vi "运维调试_总磷总氮.vi"() -> ()   [LabVIEW 2016, in "斯坦道仪器.lvlib"]
uses:
  <vilib>/Platform/TimedLoop/XDataNode/timing_clust.ctl
  <vilib>/Platform/TimedLoop/XDataNode/nitl_modes.ctl
  <vilib>/Platform/TimedLoop/XDataNode/wakeup.ctl
  <vilib>/Utility/miscctls.llb/LVPointTypeDef.ctl
  <vilib>/Utility/config.llb/Read Key (Double).vi
  <vilib>/Utility/config.llb/Write Key (Double).vi
  <vilib>/Platform/TimedLoop/XDataNode/XDataNode.xnode
  <vilib>/Platform/TimedLoop/XDataNode/XDNodeRunTimeDep.lvlib
  <vilib>/Utility/config.llb/NI_LVConfig.lvlib
panel:
  out "字符串":string
  out "总氮稀释倍数":dbl
  out "固件版本号":string
  in  "数组":string[](array[string])
  in  "备用系数写入":bool
  in  "备用系数读取":bool
  in  "备用系数":T1
  in  "量程切换阈值写入":bool
  in  "量程切换阈值读取":bool
  in  "量程切换阈值":cluster{"阈值":dbl, "标液浓度":dbl}
  in  "参数下拉列表":enum16{"总磷", "总氮"}(ring)
  in  "量程下拉列表":enum16{"低量程", "高量程"}(ring)
  in  "测量模式下拉列表":enum16{"水样测量", "空白核查", "跨度核查", "标样核查", "加标回收"}(ring)
  in  "公式":cluster{"X^2":dbl, "X":dbl, "b":dbl}
  in  "写公式":bool
  in  "读公式":bool
  in  "精度":dbl=4.0
  in  "样品5 F0":dbl
  in  "样品5 F1":dbl
  in  "样品4 F1":dbl
  in  "样品4 F0":dbl
  in  "样品3 F0":dbl
  in  "样品3 F1":dbl
  in  "样品2 F0":dbl
  in  "样品2 F1":dbl
  in  "样品1 F1":dbl
  in  "样品1 F0":dbl
  in  "method":u16(ring) items=["最小二乘", "最小绝对残差", "Bisquare"]
  in  "模型":enum32{"线性", "多项式"}(ring)
  out "r^2":dbl format="%.7g"
  out "拟合公式":string
  in  "样品2启用":bool
  in  "样品5启用":bool
  in  "样品4启用":bool
  in  "样品3启用":bool
  in  "样品1启用":bool
  in  "标液浓度5":dbl
  out "测量吸光度5":dbl
  in  "标液浓度4":dbl
  out "测量吸光度4":dbl
  in  "标液浓度3":dbl
  out "测量吸光度3":dbl
  in  "标液浓度2":dbl
  out "测量吸光度2":dbl
  out "测量吸光度1":dbl
  in  "标液浓度1":dbl
  out "XY图":cluster{"X Values":dbl[], "Y Values":dbl[]}[](graph)
  in  "返回":bool
  in  "设置":bool
  out "序列号":string="序列号"
  out "总氮测量数据":T2(xcontrol)
  out "总磷测量数据":T2(xcontrol)
  out "集成报警信息":string
  out "设置值":dbl
  out "定时启动":bool
  out "总磷总氮运行状态":T3(xcontrol)
  in  "停止":bool
  in  "手动启动":bool
  in  "单步测试":bool
  in  "总磷氨氮调试":u16[](xcontrol)
  out "F3":sgl format="%#.6f"
  out "F2":sgl format="%#.6f"
  out "F1":sgl format="%#.6f"
  out "F0":sgl format="%#.6f"
  out "多列列表框":i32(listbox)
  # "COM5"
  # "参数设置"
  # "标液浓度"
  # "F0"
  # "F1"
  # "吸光值显示"
  # "样品一"
  # "辅\n助\n计\n算\n区"
  # "样品二"
  # "样品三"
  # "样品四"
  # "样品五"
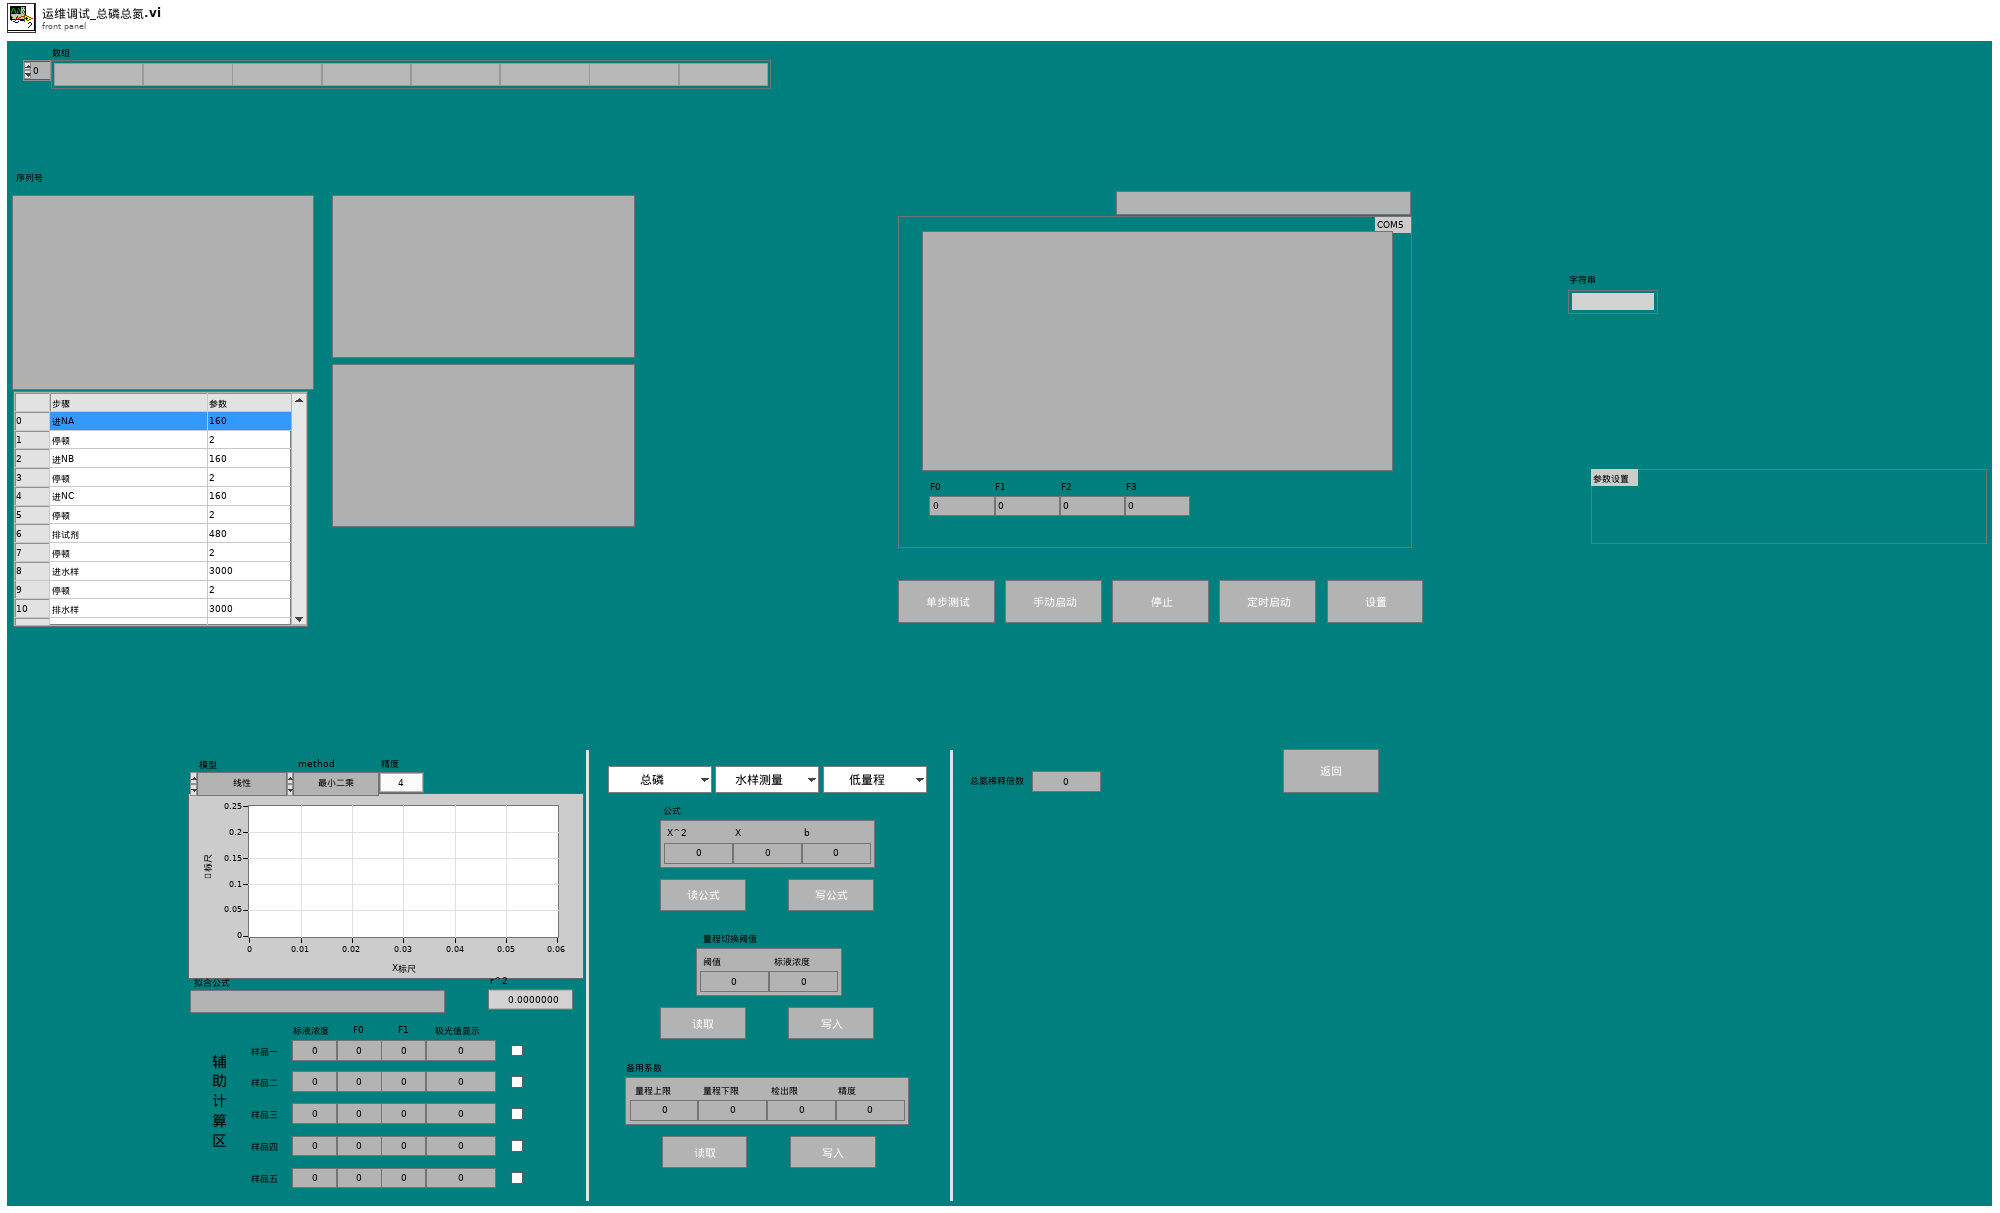
[diagram p1: front panel]
types:
  T1 = cluster{"量程上限":dbl, "量程下限":dbl, "检出限":dbl, "精度":dbl}
  T2 = cluster{"flowid":u16, "测量精度":u16, "测量数据区":cluster{"因子编码":u32, "单位":u16, "标样参考值":sgl, "水样数据时间":timestamp, "水样实测值":sgl, "水样数据标识":string, "标样数据时间":timestamp, "标样实测值":sgl, "标样数据标识":string, "空白数据时间":timestamp, "空白实测值":sgl, "空白数据标识":string, "零点核查数据时间":timestamp, "零点核查实测值":sgl, "零点核查数据标识":string, "跨度核查数据时间":timestamp, "跨度核查实测值":sgl, "跨度核查数据标识":string, "加标回收数据时间":timestamp, "加标回收实测值":sgl, "加标回收数据标识":string, "平行样数据时间":timestamp, "平行样实测值":sgl, "平行样数据标识":string, "F0":sgl, "F1":sgl, "F2":sgl, "F3":sgl, "F4":sgl, "F5":sgl, "F6":sgl, "F7":sgl, "温度":sgl, "湿度":sgl, "X值":sgl}}
  T3 = cluster{"系统时间":timestamp, "工作状态":enum16{"空闲", "水样测试", "标样核查", "零点核查", "跨度核查", "空白测试", "平行样测试", "加标回收", "空白校准", "标样校准", "初始化（清洗）"}, "测量模式":enum16{"待机", "连续模式", "周期模式", "定点模式", "受控模式", "手动模式"}, "告警代码":enum16{"无告警", "缺试剂告警", "缺水样告警", "缺蒸馏水告警", "缺标液告警", "仪表漏液告警", "标定异常告警", "超量程告警", "加热异常", "低试剂预警", "超上限告警", "超下限告警", "仪表内部其他异常", "滴定异常告警", "电极异常告警", "量程切换告警", "参数设置告警", "PH电极电位异常", "电导率电极异常", "浊度光度异常", "溶解氧电极异常", "溶解氧光强异常", "温度异常告警", "PH异常告警", "溶解氧异常告警", "电导率异常告警", "浊度异常告警", "叶绿素异常告警", "藻密度异常告警", "蓝绿藻异常告警", "ORP异常告警", "氨氮异常告警", "清洁刷异常告警", "SD卡异常告警", "蓝牙异常告警", "Wifi异常告警", "流程异常告警"}, "故障代码":enum16{"无故障", "电机故障", "温度故障", "通讯故障", "滴定故障"}, "日志代码":u16, "软件版本":u16, "F0":sgl, "F1":sgl, "F2":sgl, "F3":sgl, "T":sgl, "H":sgl, "id":u16, "flowid":u16, "量程":u16}
  T4 = enum16{"待机", "启动氨氮", "氨氮测量中", "启动总磷", "总磷测量中", "延时"}
  T5 = typedef "LVPointTypeDef.ctl" = cluster{"Horizontal":i16, "Vertical":i16}
  T6 = cluster{"因子编码":u32, "单位":u16, "标样参考值":sgl, "水样数据时间":timestamp, "水样实测值":sgl, "水样数据标识":string, "标样数据时间":timestamp, "标样实测值":sgl, "标样数据标识":string, "空白数据时间":timestamp, "空白实测值":sgl, "空白数据标识":string, "零点核查数据时间":timestamp, "零点核查实测值":sgl, "零点核查数据标识":string, "跨度核查数据时间":timestamp, "跨度核查实测值":sgl, "跨度核查数据标识":string, "加标回收数据时间":timestamp, "加标回收实测值":sgl, "加标回收数据标识":string, "平行样数据时间":timestamp, "平行样实测值":sgl, "平行样数据标识":string, "F0":sgl, "F1":sgl, "F2":sgl, "F3":sgl, "F4":sgl, "F5":sgl, "F6":sgl, "F7":sgl, "温度":sgl, "湿度":sgl, "X值":sgl}
  T7 = enum16{"空闲", "水样测试", "标样核查", "零点核查", "跨度核查", "空白测试", "平行样测试", "加标回收", "空白校准", "标样校准", "初始化（清洗）"}
  T8 = typedef "XDNodeRunTimeDep.lvlib/timing_clust.ctl" = cluster{"Expected End [f-1]":u64, "Actual End [f-1]":u64, "Finished Late? [f-1]":bool, "Expected End [i-1]":u64, "Actual End [i-1]":u64, "Finished Late? [i-1]":bool, "Expected Start [i]":u64, "Actual Start [i]":u64, "Expected Start [f]":u64, "Actual Start [f]":u64, "Source Name":string, "Structure Name":string, "Period":i64, "Deadline":i64, "Offset":i64, "Start":i64, "Priority":i32, "Timeout":i32, "Mode":T9, "Wakeup Reason":T10, "Error":errorcluster, "Source Type":string, "Secondary Source Type":string, "Global End Time":u64, "Global Start Time":u64, "Frame Duration":u64, "Iteration Duration":u64, "Assigned CPU":i32, "I/O Scan Engine Mode":u32}
  T9 = typedef "XDNodeRunTimeDep.lvlib/nitl_modes.ctl" = enum32{"No Change", "Process missed periods, maintain original phase", "Discard missed periods, maintain original phase", "Process missed periods, ignore original phase", "Discard missed periods, ignore original phase"}
  T10 = typedef "XDNodeRunTimeDep.lvlib/wakeup.ctl" = enum32{"Normal", "Aborted", "Asynchronous wakeup", "Timing source error", "Timed loop error", "Timeout"}
  T11 = cluster{"启动模式":enum16{"标液测量", "水样测量", "零液测量", "盲样测量", "加标回收"}, "启动参数":u16, "量程":enum16{"低量程", "高量程"}}
  T12 = cluster{"时间标识":timestamp, "设备":string, "日志信息":string, "流程参数":string}
  T13 = cluster{"时间标识":timestamp, "设备":string, "日志信息":string}
  T14 = enum16{"无告警", "缺试剂告警", "缺水样告警", "缺蒸馏水告警", "缺标液告警", "仪表漏液告警", "标定异常告警", "超量程告警", "加热异常", "低试剂预警", "超上限告警", "超下限告警", "仪表内部其他异常", "滴定异常告警", "电极异常告警", "量程切换告警", "参数设置告警", "PH电极电位异常", "电导率电极异常", "浊度光度异常", "溶解氧电极异常", "溶解氧光强异常", "温度异常告警", "PH异常告警", "溶解氧异常告警", "电导率异常告警", "浊度异常告警", "叶绿素异常告警", "藻密度异常告警", "蓝绿藻异常告警", "ORP异常告警", "氨氮异常告警", "清洁刷异常告警", "SD卡异常告警", "蓝牙异常告警", "Wifi异常告警", "流程异常告警"}
  T15 = typedef "LVRowAndColumnUnsignedTypeDef.ctl" = cluster{"Row":u32, "Column":u32}
  T16 = typedef "NI_LVConfig.lvlib/Config Data RefNum.ctl" = refnum<k1>
  T17 = cluster{"站号":u16, "量程切换":enum32{"H", "L", "AUTO"}, "控制命令":enum16{"启动测量", "标样核查", "零点核查", "跨度核查", "空白测试", "平行样测试", "加标回收", "空白校准", "标样校准", "初始化（清洗）", "停止测试", "仪器重启", "校时", "模式设置", "测量间隔设置", "盲样测试"}, "模式设置":enum16{"待机", "连续模式", "周期模式", "定点模式", "受控模式", "手动模式"}, "测量间隔":u16}
  T18 = cluster{"站号":u16, "量程切换":enum32{"H", "L", "AUTO"}, "控制命令":enum16{"启动测量", "标样核查", "零点核查", "跨度核查", "空白测试", "平行样测试", "加标回收", "空白校准", "标样校准", "初始化（清洗）", "停止测试", "仪器重启", "校时", "模式设置", "测量间隔设置"}, "模式设置":enum16{"待机", "连续模式", "周期模式", "定点模式", "受控模式", "手动模式"}, "测量间隔":u16}
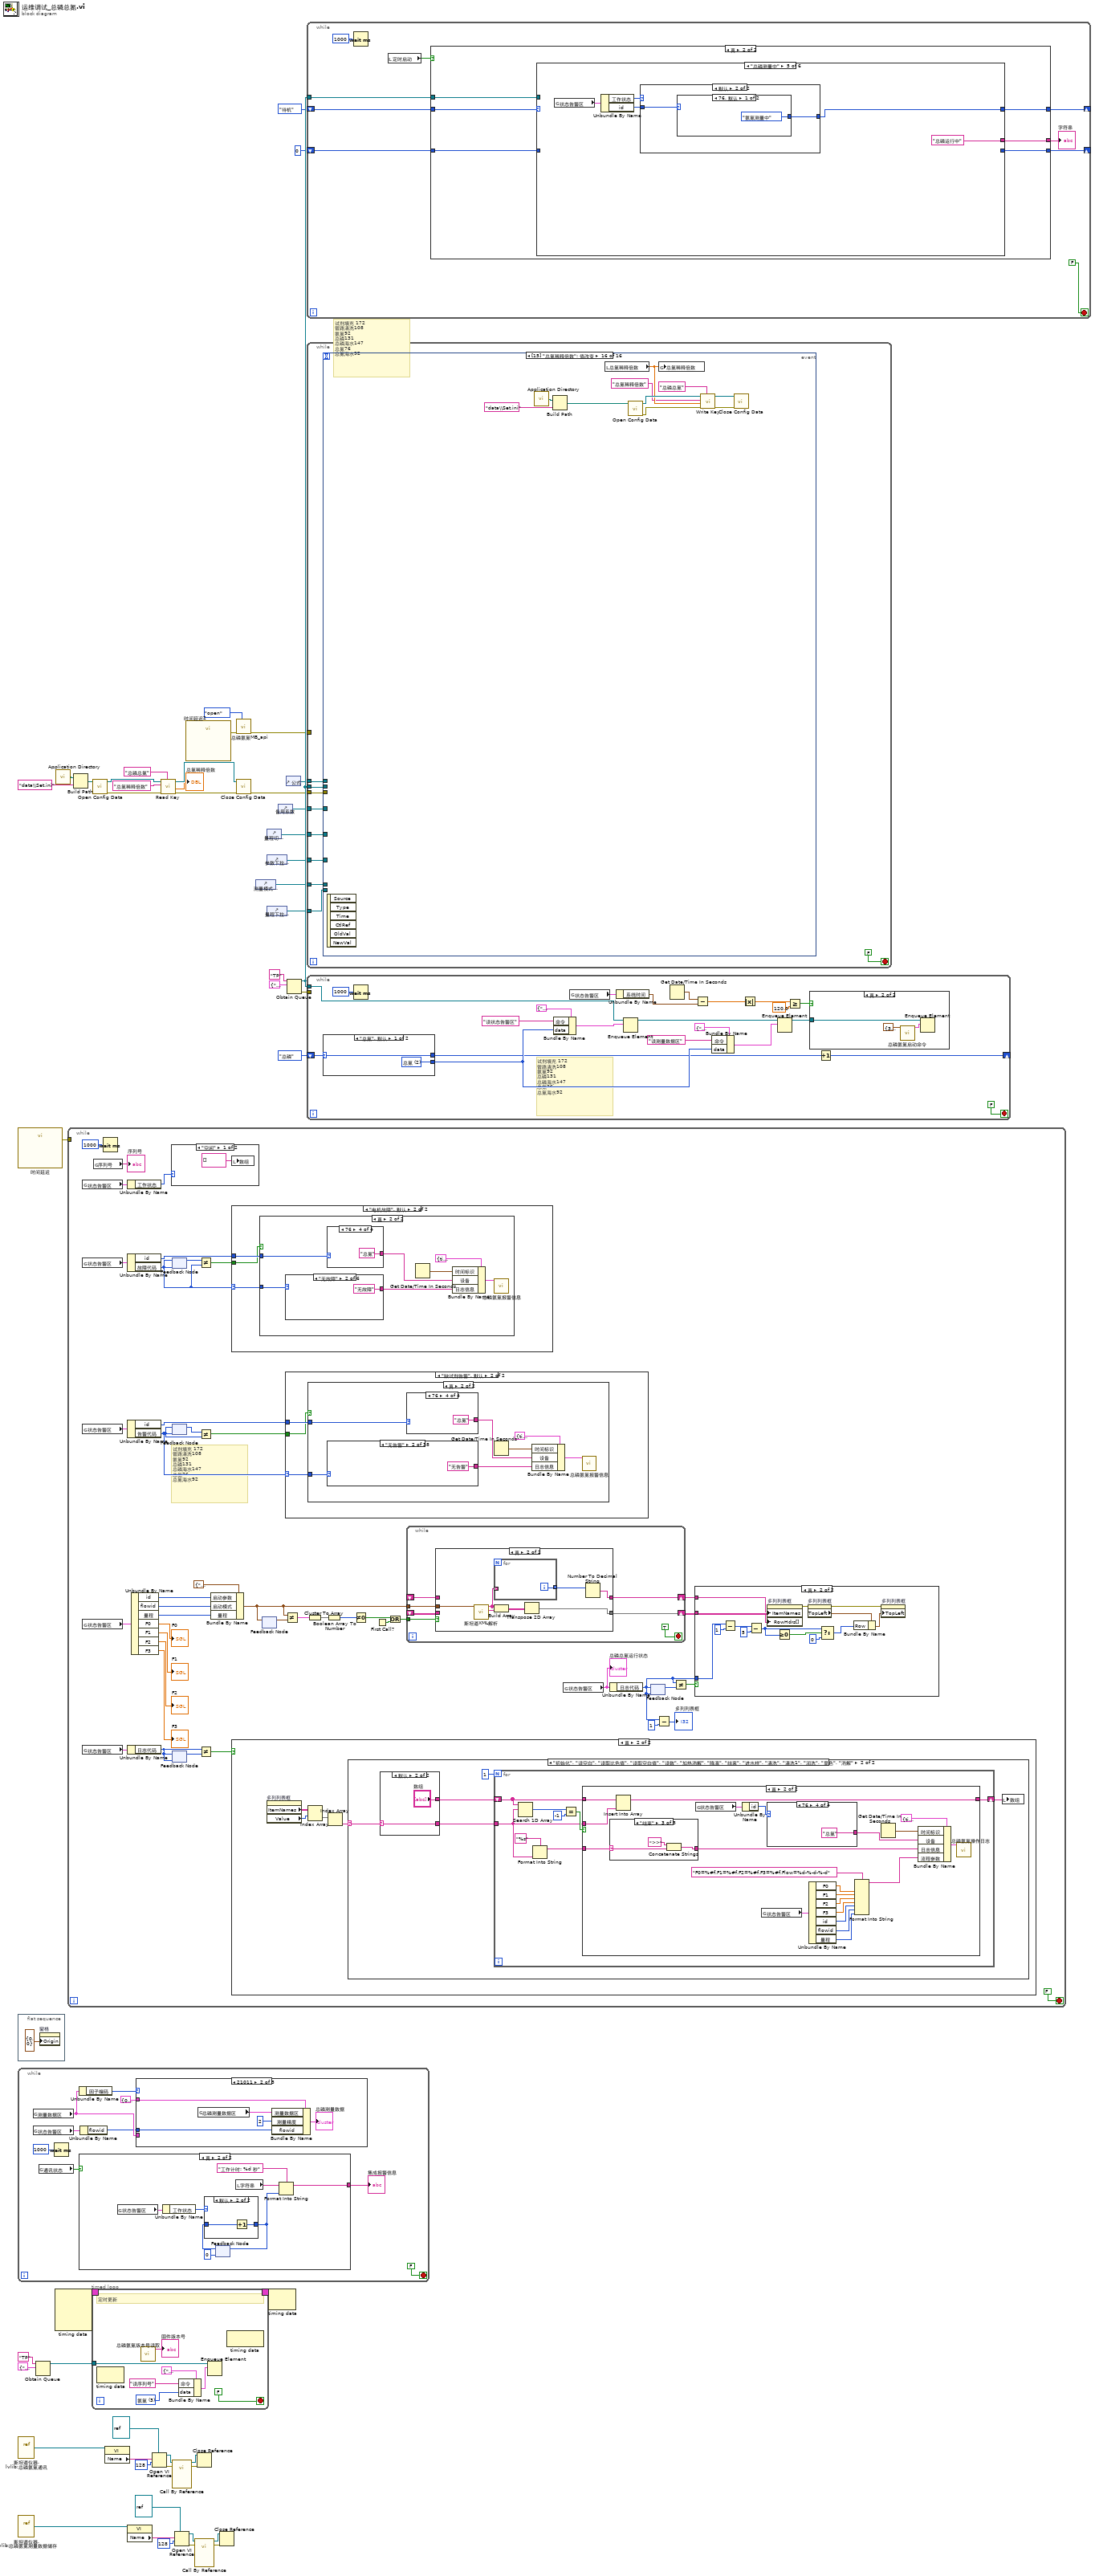
[diagram p0: block diagram]
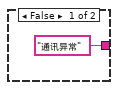
[diagram p2: hidden frame]
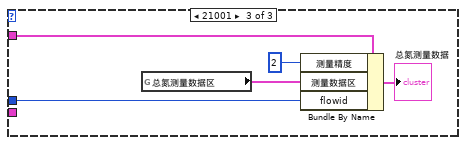
[diagram p5: hidden frame]
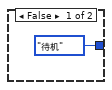
[diagram p6: hidden frame]
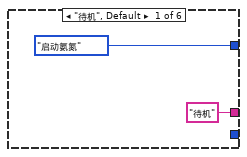
[diagram p7: hidden frame]
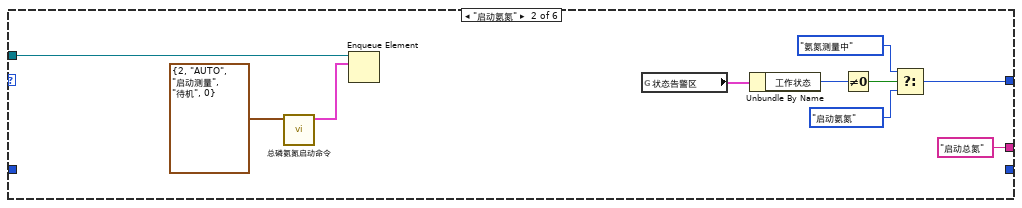
[diagram p8: hidden frame]
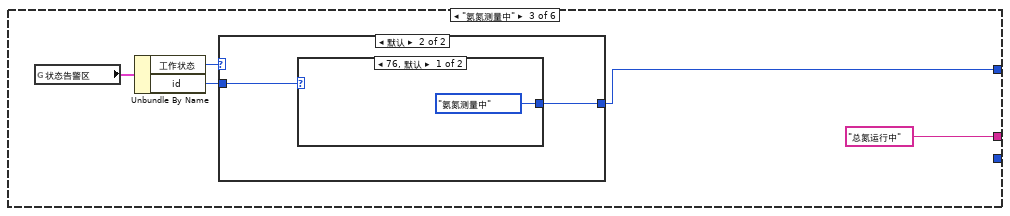
[diagram p9: hidden frame]
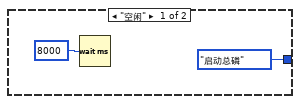
[diagram p10: hidden frame]
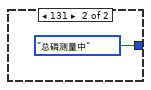
[diagram p11: hidden frame]
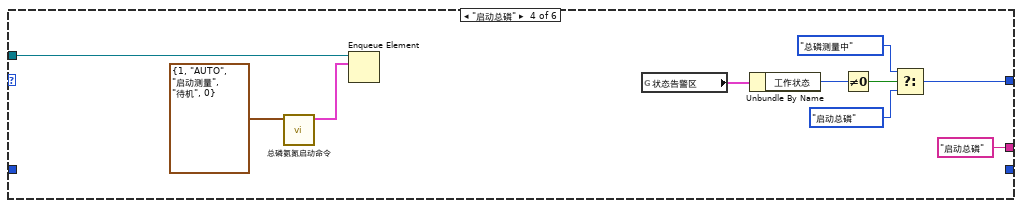
[diagram p12: hidden frame]
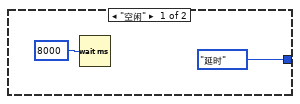
[diagram p13: hidden frame]
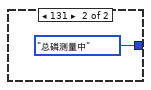
[diagram p14: hidden frame]
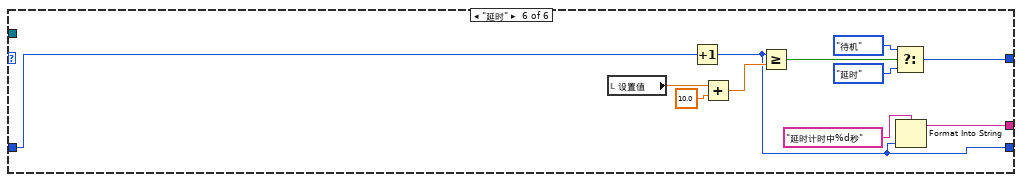
[diagram p15: hidden frame]
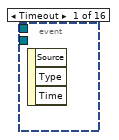
[diagram p16: hidden frame]
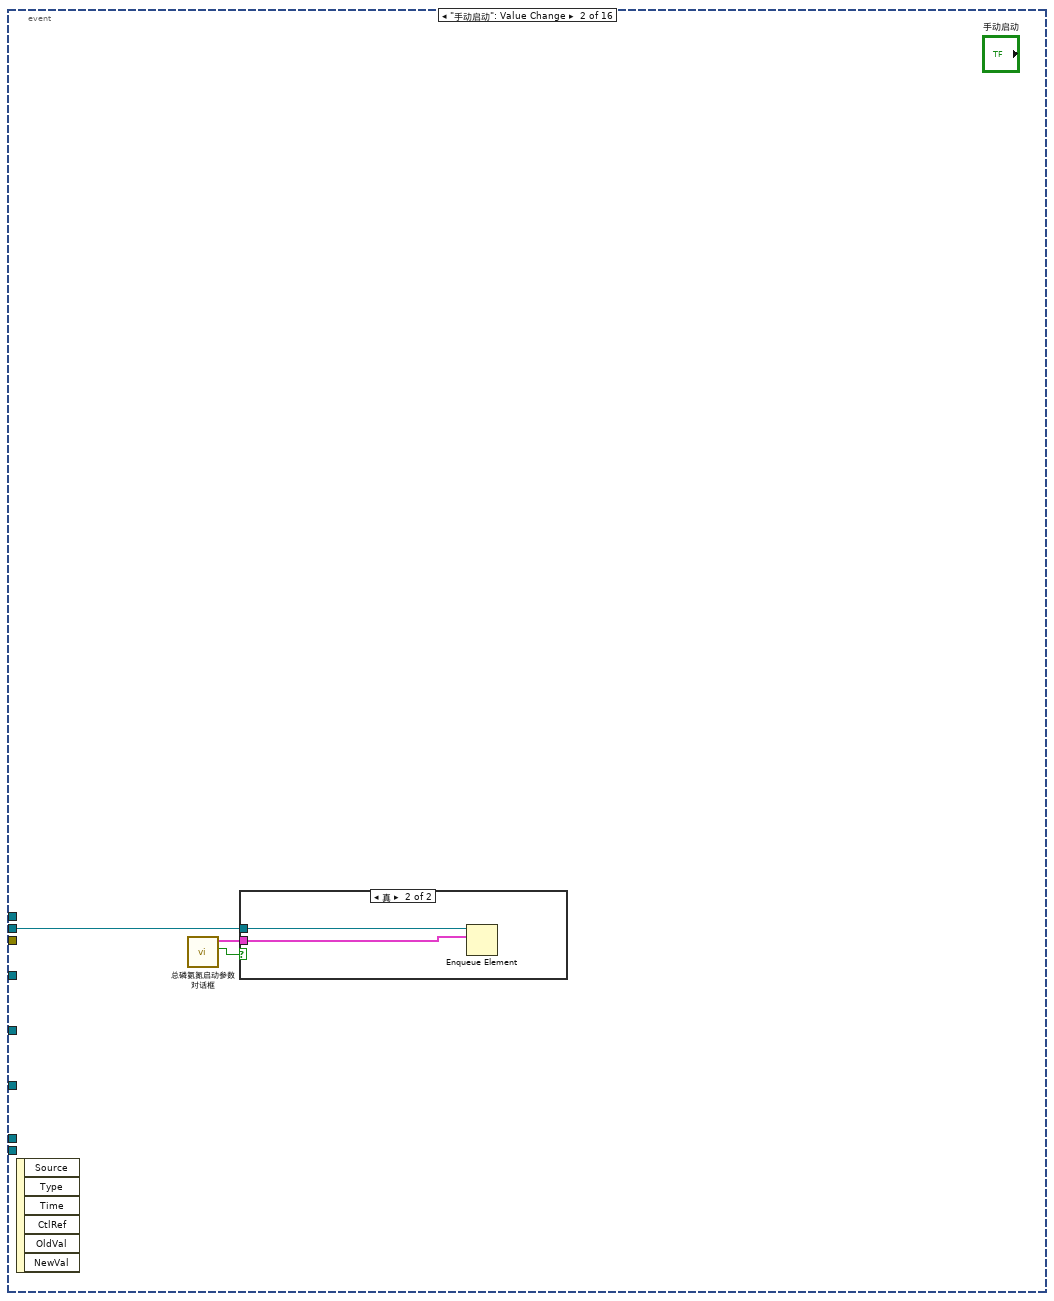
[diagram p17: hidden frame]
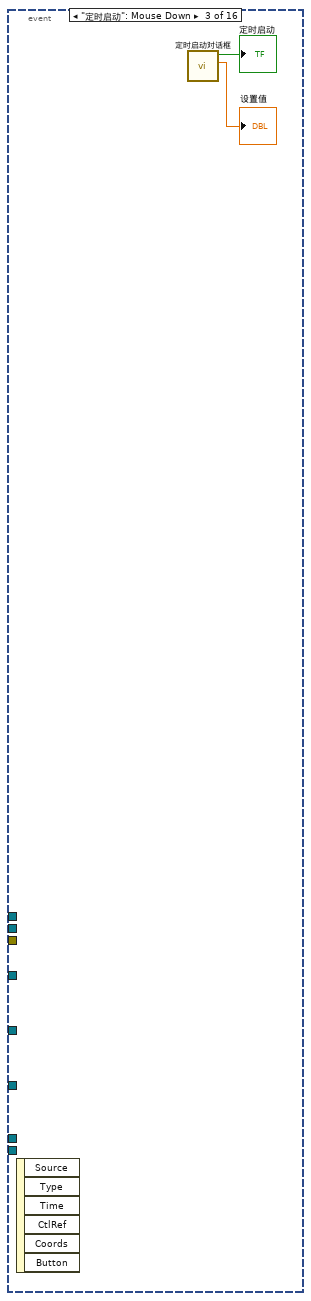
[diagram p19: hidden frame]
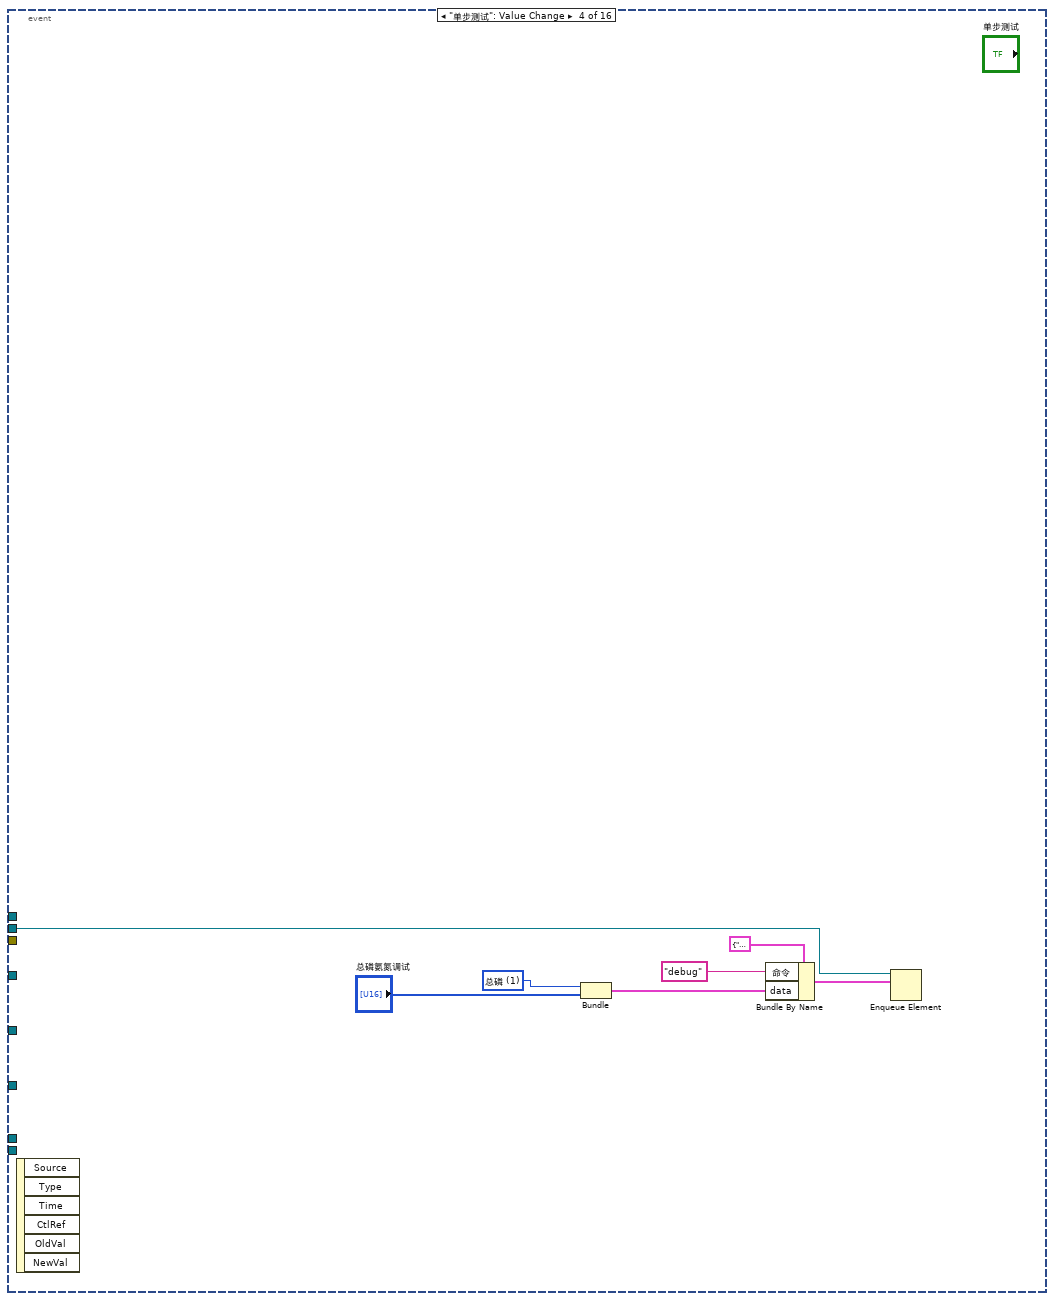
[diagram p20: hidden frame]
diagram:
  # "试剂填充 172 \n管路清洗108\n氨氮92\n总磷131\n总磷海水147\n总氮76\n总氮海水92"
  n1 = call "时间延迟"() -> ("error out"=w20:errorcluster)  [unwired: 11 in]
  n2 = flat-sequence {
    frame #0 {
      n3 = property on="窗格" class="Pane"("Origin"=T5 {"Horizontal"=0, "Vertical"=0} ("原点")) -> ()  [unwired: 2 in, 2 out]
    }
  }
  n4 = while {
    stop <- FALSE stop-if-true
    n5 = global read "VAR总磷氨氮全局变量.vi" "测量数据区"() -> (w57:T6)
    n6 = global read "VAR总磷氨氮全局变量.vi" "状态告警区"() -> (w53:T3)
    n7 = global read "VAR总磷氨氮全局变量.vi" "通讯状态"() -> (w55:bool)
    n8 = Wait (ms)(milliseconds to wait=u32 1000 ("等待时间（毫秒）")) -> ()  [unwired: 1 out]
    n9 = Unbundle By Name(w57) -> ("因子编码"=w56:u32)
    n10 = case shown="真" w55 {
      tunnel: ["通讯异常" ("集成报警信息") w62] -> w54
      frame False {
      }
      frame True {
        n11 = global read "VAR总磷氨氮全局变量.vi" "状态告警区"() -> (w68:T3)
        n12 = Unbundle By Name(w68) -> ("工作状态"=w67:T7)
        n13 = feedback #1(0) -> (w65:i32)
        n14 = case shown="默认" w67 {
          tunnel: w65 -> [_ w70]
          tunnel: [_ w69] -> w63
          frame "空闲" {
          }
          frame Default {
            n15 = Increment(x=w70) -> (x+1=w69:i32)
          }
        }
        n16 = feedback-in #1(w63) -> ()
        n17 = local read "字符串"() -> (w61:string)
        n18 = Format Into String(format string="工作计时: %d 秒" ("格式字符串"), initial string=w61, w63) -> (resulting string=w62:string)  [unwired: 1 in, 1 out]
      }
    }
    "集成报警信息" <- w54
    n19 = Unbundle By Name(w53) -> ("flowid"=w52:u16)
    n20 = case shown="21011" w56 {
      tunnel: w57 -> [_ _ _]
      tunnel: w52 -> [_ w73 w79]
      tunnel: T2 {"flowid"=0, "测量精度"=0, "测量数据区"={"因子编码"=0, "单位"=0, "标样参考值"=0.0, "水样数据时间"=timestamp(0 s since 1904-01-01), "水样实测值"=0.0, "水样数据标识"="", "标样数据时间"=timestamp(0 s since 1904-01-01), "标样实测值"=0.0, "标样数据标识"="", "空白数据时间"=timestamp(0 s since 1904-01-01), "空白实测值"=0.0, "空白数据标识"="", "零点核查数据时间"=timestamp(0 s since 1904-01-01), "零点核查实测值"=0.0, "零点核查数据标识"="", "跨度核查数据时间"=timestamp(0 s since 1904-01-01), "跨度核查实测值"=0.0, "跨度核查数据标识"="", "加标回收数据时间"=timestamp(0 s since 1904-01-01), "加标回收实测值"=0.0, "加标回收数据标识"="", "平行样数据时间"=timestamp(0 s since 1904-01-01), "平行样实测值"=0.0, "平行样数据标识"="", "F0"=0.0, "F1"=0.0, "F2"=0.0, "F3"=0.0, "F4"=0.0, "F5"=0.0, "F6"=0.0, "F7"=0.0, "温度"=0.0, "湿度"=0.0, "X值"=0.0}} ("总氮测量数据") -> [_ w72 w78]
      frame Default {
      }
      frame 21011 {
        n21 = global read "VAR总磷氨氮全局变量.vi" "总磷测量数据区"() -> (w71:T6)
        n22 = Bundle By Name(cluster=w72, "测量数据区"=w71, "测量精度"=u16 2, "flowid"=w73) -> (→"总磷测量数据":T2)
      }
      frame 21001 {
        n23 = global read "VAR总磷氨氮全局变量.vi" "总氮测量数据区"() -> (w76:T6)
        n24 = Bundle By Name(cluster=w78, "测量精度"=u16 2, "测量数据区"=w76, "flowid"=w79) -> (→"总氮测量数据":T2)
      }
    }
  }
  n25 = vi-ref "斯坦道仪器.lvlib:总磷氨氮通讯.vi"() -> (w43:refnum<vi>)
  n26 = vi-ref "斯坦道仪器.lvlib:总磷氨氮测量数据储存.vi"() -> (w35:refnum<vi>)
  n27 = Obtain Queue(name (unnamed)="TP" ("名称（未命名）"), element data type=cluster{"命令":string, "data":variant} {"命令"="", "data"=variant}) -> (queue out=w13:refnum<queue>)  [unwired: 3 in, 2 out]
  n28 = node-c288() -> (w17:T8)  [unwired: 4 in]
  n29 = call <vilib>:"Application Directory.vi"() -> ("Application Directory"=w7:path)
  n30 = while {
    tunnel: w20 -> [_]
    stop <- FALSE stop-if-true
    # "试剂填充 172 \n管路清洗108\n氨氮92\n总磷131\n总磷海水147\n总氮76\n总氮海水92"
    n31 = global read "VAR总磷氨氮全局变量.vi" "状态告警区"() -> (w89:T3)
    n32 = global read "VAR总磷氨氮全局变量.vi" "状态告警区"() -> (w94:T3)
    n33 = global read "VAR总磷氨氮全局变量.vi" "状态告警区"() -> (w99:T3)
    n34 = global read "VAR总磷氨氮全局变量.vi" "状态告警区"() -> (w111:T3)
    n35 = global read "VAR总磷氨氮全局变量.vi" "状态告警区"() -> (w86:T3)
    n36 = global read "VAR总磷氨氮全局变量.vi" "序列号"() -> (→"序列号":string)
    n37 = Wait (ms)(milliseconds to wait=u32 1000 ("等待时间（毫秒）")) -> ()  [unwired: 1 out]
    n38 = Unbundle By Name(w89) -> ("工作状态"=w88:T7)
    n39 = Unbundle By Name(w94) -> ("id"=w93:u16, "故障代码"=w90:enum16{"无故障", "电机故障", "温度故障", "通讯故障", "滴定故障"})
    n40 = Unbundle By Name(w99) -> ("id"=w98:u16, "告警代码"=w95:T14)
    n41 = Unbundle By Name(w86) -> ("日志代码"=w85:u16)
    n42 = Unbundle By Name(w111) -> ("id"=w108:u16, "flowid"=w110:u16, "量程"=w109:u16, "F0"=→"F0":sgl, "F1"=→"F1":sgl, "F2"=→"F2":sgl, "F3"=→"F3":sgl)
    n43 = case shown="\"空闲\"" w88 {
      frame "空闲" {
        n44 = local write "数组"(string[] [] ("数组")) -> ()
      }
      frame "水样测试", Default {
      }
    }
    n45 = feedback #2(w90) -> (w91:enum16{"无故障", "电机故障", "温度故障", "通讯故障", "滴定故障"})
    n46 = feedback-in #2(w90) -> ()
    n47 = feedback #3(w95) -> (w96:T14)
    n48 = feedback-in #3(w95) -> ()
    n49 = feedback #4(w85) -> (w87:u16)
    n50 = feedback-in #4(w85) -> ()
    n51 = Not Equal?(x=w91, y=w90) -> (x != y?=w92:bool)
    n52 = Not Equal?(x=w96, y=w95) -> (x != y?=w97:bool)
    n53 = Not Equal?(x=w85, y=w87) -> (x != y?=w84:bool)
    n54 = Bundle By Name(cluster=T11 {"启动模式"=enum."加标回收", "启动参数"=1, "量程"=enum."低量程"} ("参数簇"), "启动参数"=w108, "启动模式"=w110, "量程"=w109) -> (w101:T11)
    n55 = case shown="\"电机故障\", 默认" w90 {
      selector: w90 -> [_ w180]
      tunnel: w93 -> [_ w181]
      tunnel: w92 -> [_ w179]
      frame "无故障" {
      }
      frame "电机故障", Default {
        n56 = case shown="真" w179 {
          tunnel: w181 -> [_ w188]
          tunnel: w180 -> [_ w183]
          frame False {
          }
          frame True {
            n57 = case shown="\"无故障\"" w183 {
              selector: w183 -> [w190 _ _ _ _ _]
              tunnel: [w189 "无故障" "电机故障" "温度故障" "通讯故障" "滴定故障"] -> w182
              frame Default {
                n58 = Format Into String(format string="%d" ("格式字符串"), initial string="未知" ("工作状态"), w190) -> (resulting string=w189:string)  [unwired: 1 in, 1 out]
              }
              frame "无故障" {
              }
              frame "电机故障" {
              }
              frame "温度故障" {
              }
              frame "通讯故障" {
              }
              frame "滴定故障" {
              }
            }
            n59 = case shown="76" w188 {
              tunnel: [_ "总磷" ("table输入") "氨氮" ("table输入") "总氮" ("table输入")] -> w184
              frame Default {
              }
              frame 131 {
              }
              frame 92 {
              }
              frame 76 {
              }
            }
            n60 = Get Date/Time In Seconds() -> (seconds since 1Jan1904=w185:timestamp)
            n61 = Bundle By Name(cluster=T13 {"时间标识"=timestamp(0 s since 1904-01-01), "设备"="", "日志信息"=""} ("data in"), "时间标识"=w185, "设备"=w184, "日志信息"=w182) -> (w186:T13)
            n62 = call "总磷氨氮报警信息.vi"("data in"=w186) -> ()  [unwired: 11 in]
          }
        }
      }
    }
    n63 = case shown="真" w84 {
      frame False {
      }
      frame True {
        n64 = property on="多列列表框" class="MCListbox (严格)"() -> ("ItemNames"=w128:string[][], "Value"=w129:i32)  [unwired: 2 in, 2 out]
        n65 = Index Array(array=w128, index (row)=w129) -> (element=w127:string[])  [unwired: 1 in]
        n66 = Index Array(array=w127) -> (element=w126:string)  [unwired: 1 in]
        n67 = case shown="\"初始化\", \"读空白\", \"读取比色值\", \"读取空白值\", \"读数\", \"加热消解\", \"降温\", \"结束\", \"进水样\", \"清洗\", \"清洗1\", \"润洗\", \"显色\", \"消解\"" w126 {
          selector: w126 -> [_ w132]
          frame Default {
          }
          frame "初始化", "读空白", "读取比色值", "读取空白值", "读数", "加热消解", "降温", "结束", "进水样", "清洗", "清洗1", "润洗", "显色", "消解" {
            n68 = case shown="默认" w132 {
              selector: w132 -> [w136 w138]
              tunnel: [w136 w138] -> w131
              tunnel: [string[] [] ("数组") "数组"] -> w130
              frame "读数" {
              }
              frame Default {
              }
            }
            n69 = for {
              N: 1 -> [_]
              tunnel: w131 -> [w140]
              shift-right: [w139] -> w133
              shift-left: w130 -> [w141]
              n70 = Search 1D Array(1D array=w141, element=w140) -> (index of element=w144:i32)  [unwired: 1 in]
              n71 = Format Into String(format string="%s" ("格式字符串"), w140) -> (resulting string=w145:string)  [unwired: 2 in, 1 out]
              n72 = Equal?(x=w144, y=-1) -> (x = y?=w142:bool)
              n73 = case shown="真" w142 {
                tunnel: w145 -> [_ w149]
                tunnel: w141 -> [w147 w153]
                tunnel: w140 -> [_ w152]
                tunnel: [w147 w151] -> w139
                frame False {
                }
                frame True {
                  n74 = case shown="\"结束\"" w149 {
                    selector: w149 -> [w169 w172 w175]
                    tunnel: [w169 w171 w174] -> w148
                    frame Default {
                    }
                    frame "初始化" {
                      n75 = Concatenate Strings("<<" ("字符串"), w172) -> (w171:string)
                    }
                    frame "结束" {
                      n76 = Concatenate Strings(">>" ("字符串"), w175) -> (w174:string)
                    }
                  }
                  n77 = Insert Into Array(array=w153, new element=w152) -> (w151:string[])  [unwired: 1 in]
                  n78 = global read "VAR总磷氨氮全局变量.vi" "状态告警区"() -> (w168:T3)
                  n79 = Unbundle By Name(w168) -> ("id"=w167:u16)
                  n80 = global read "VAR总磷氨氮全局变量.vi" "状态告警区"() -> (w163:T3)
                  n81 = case shown="76" w167 {
                    tunnel: [_ "总磷" ("table输入") "氨氮" ("table输入") "总氮" ("table输入")] -> w165
                    frame Default {
                    }
                    frame 131 {
                    }
                    frame 92 {
                    }
                    frame 76 {
                    }
                  }
                  n82 = Unbundle By Name(w163) -> ("F0"=w160:sgl, "F1"=w159:sgl, "F2"=w158:sgl, "F3"=w157:sgl, "id"=w156:u16, "flowid"=w155:u16, "量程"=w154:u16)
                  n83 = Format Into String(format string="F0=%#f,F1=%#f,F2=%#f,F3=%#f,Flow=%d-%-d-%-d" ("格式字符串"), w160, w159, w158, w157, w156, w155, w154) -> (resulting string=w161:string)  [unwired: 2 in, 1 out]
                  n84 = Get Date/Time In Seconds() -> (seconds since 1Jan1904=w164:timestamp)
                  n85 = Bundle By Name(cluster=T12 {"时间标识"=timestamp(0 s since 1904-01-01), "设备"="", "日志信息"="", "流程参数"=""} ("data in"), "时间标识"=w164, "设备"=w165, "日志信息"=w148, "流程参数"=w161) -> (w166:T12)
                  n86 = call "总磷氨氮操作日志.vi"("data in"=w166) -> ()  [unwired: 11 in]
                }
              }
            }
            n87 = local write "数组"(w133) -> ()
          }
        }
      }
    }
    n88 = feedback #5() -> (w117:T11)  [unwired: 1 in]
    n89 = feedback-in #5(w101) -> ()
    n90 = Not Equal?(x=w101, y=w117) -> (x != y?=w118:cluster{"启动模式":bool, "启动参数":bool, "量程":bool})
    n91 = case shown="\"缺试剂告警\", 默认" w95 {
      selector: w95 -> [_ w202]
      tunnel: w98 -> [_ w203]
      tunnel: w97 -> [_ w201]
      frame "无告警" {
      }
      frame "缺试剂告警", Default {
        n92 = case shown="真" w201 {
          tunnel: w203 -> [_ w210]
          tunnel: w202 -> [_ w204]
          frame False {
          }
          frame True {
            n93 = case shown="\"无告警\"" w204 {
              selector: w204 -> [w212 _ _ _ _ _ _ _ _ _ _ _ _ _ _ _ _ _ _ _ _ _ _ _ _ _ _ _ _ _ _ _ _ _ _ _ _ _]
              tunnel: [w211 "无告警" "缺试剂告警" "缺水样告警" "缺蒸馏水告警" "缺标液告警" "仪表漏液告警" "标定异常告警" "超量程告警" "加热异常" "低试剂预警" "超上限告警" "超下限告警" "仪表内部其他异常" "滴定异常告警" "电极异常告警" "量程切换告警" "参数设置告警" "PH电极电位异常" "电导率电极异常" "浊度光度异常" "溶解氧电极异常" "溶解氧光强异常" "温度异常告警" "PH异常告警" "溶解氧异常告警" "电导率异常告警" "浊度异常告警" "叶绿素异常告警" "藻密度异常告警" "蓝绿藻异常告警" "ORP异常告警" "氨氮异常告警" "清洁刷异常告警" "SD卡异常告警" "蓝牙异常告警" "WiFi异常告警" "流程异常告警"] -> w205
              frame Default {
                n94 = Format Into String(format string="%d" ("格式字符串"), initial string="未知" ("工作状态"), w212) -> (resulting string=w211:string)  [unwired: 1 in, 1 out]
              }
              frame "无告警" {
              }
              frame "缺试剂告警" {
              }
              frame "缺水样告警" {
              }
              frame "缺蒸馏水告警" {
              }
              frame "缺标液告警" {
              }
              frame "仪表漏液告警" {
              }
              frame "标定异常告警" {
              }
              frame "超量程告警" {
              }
              frame "加热异常" {
              }
              frame "低试剂预警" {
              }
              frame "超上限告警" {
              }
              frame "超下限告警" {
              }
              frame "仪表内部其他异常" {
              }
              frame "滴定异常告警" {
              }
              frame "电极异常告警" {
              }
              frame "量程切换告警" {
              }
              frame "参数设置告警" {
              }
              frame "PH电极电位异常" {
              }
              frame "电导率电极异常" {
              }
              frame "浊度光度异常" {
              }
              frame "溶解氧电极异常" {
              }
              frame "溶解氧光强异常" {
              }
              frame "温度异常告警" {
              }
              frame "PH异常告警" {
              }
              frame "溶解氧异常告警" {
              }
              frame "电导率异常告警" {
              }
              frame "浊度异常告警" {
              }
              frame "叶绿素异常告警" {
              }
              frame "藻密度异常告警" {
              }
              frame "蓝绿藻异常告警" {
              }
              frame "ORP异常告警" {
              }
              frame "氨氮异常告警" {
              }
              frame "清洁刷异常告警" {
              }
              frame "SD卡异常告警" {
              }
              frame "蓝牙异常告警" {
              }
              frame "Wifi异常告警" {
              }
              frame "流程异常告警" {
              }
            }
            n95 = case shown="76" w210 {
              tunnel: [_ "总磷" ("table输入") "氨氮" ("table输入") "总氮" ("table输入")] -> w206
              frame Default {
              }
              frame 131 {
              }
              frame 92 {
              }
              frame 76 {
              }
            }
            n96 = Get Date/Time In Seconds() -> (seconds since 1Jan1904=w207:timestamp)
            n97 = Bundle By Name(cluster=T13 {"时间标识"=timestamp(0 s since 1904-01-01), "设备"="", "日志信息"=""} ("data in"), "时间标识"=w207, "设备"=w206, "日志信息"=w205) -> (w208:T13)
            n98 = call "总磷氨氮报警信息.vi"("data in"=w208) -> ()  [unwired: 11 in]
          }
        }
      }
    }
    n99 = Cluster To Array(cluster=w118) -> (array=w119:bool[])
    n100 = Boolean Array To Number(Boolean array=w119) -> (number=w120:u32)
    n101 = Not Equal To 0?(x=w120) -> (x != 0?=w113:bool)
    n102 = First Call?() -> (First Call?: T/F=w114:bool)
    n103 = Or(x=w113, y=w114) -> (x .or. y?=w112:bool)
    n104 = while {
      tunnel: w112 -> [w261]
      tunnel: w101 -> [w260]
      shift-right: [w259] -> w116
      shift-left: _ -> [w255]
      shift-right: [w258] -> w115
      shift-left: _ -> [w256]
      stop <- TRUE stop-if-true
      n105 = case shown="真" w261 {
        tunnel: [w263 w270] -> w258
        tunnel: [w262 w269] -> w259
        tunnel: w260 -> [_ w264]
        tunnel: w256 -> [w263 _]
        tunnel: w255 -> [w262 _]
        frame False {
        }
        frame True {
          n106 = call "斯坦道XML解析.vi"("参数簇"=w264) -> ("步骤时间"=w265:string[], "步骤名"=w267:string[])  [unwired: 9 in]
          n107 = for {
            tunnel: w267 -> [_] mode=indexing
            tunnel: [w271] -> w268 mode=indexing
            i -> [w271]
          }
          n108 = Build Array(w267, w265) -> (w266:string[][])
          n109 = Transpose 2D Array(2D array=w266) -> (transposed array=w269:string[][])
          n110 = Number To Decimal String(number=w268) -> (decimal integer string=w270:string[])  [unwired: 1 in]
        }
      }
    }
    n111 = global read "VAR总磷氨氮全局变量.vi" "状态告警区"() -> (w102:T3)
    "总磷总氮运行状态" <- w102
    n112 = Unbundle By Name(w102) -> ("日志代码"=w82:u16)
    n113 = feedback-in #6(w82) -> ()
    n114 = feedback #6(w82) -> (w122:u16)
    n115 = Subtract(x=w82, y=1) -> (x-y=→"多列列表框":i32)
    n116 = Not Equal?(x=w82, y=w122) -> (x != y?=w121:bool)
    n117 = case shown="真" w121 {
      tunnel: w82 -> [_ w274]
      tunnel: w116 -> [_ w281]
      tunnel: w115 -> [_ w280]
      frame False {
      }
      frame True {
        n118 = Subtract(x=w274, y=1) -> (x-y=w272:i32)
        n119 = Subtract(x=w272, y=5) -> (x-y=w276:i32)
        n120 = property on="多列列表框" class="MCListbox (严格)"("ItemNames"=w281, "RowHdrs[]"=w280) -> (error out=w282:errorcluster)  [unwired: 2 in, 1 out]
        n121 = Greater Or Equal To 0?(x=w276) -> (x >= 0?=w275:bool)
        n122 = property on="多列列表框" class="MCListbox (严格)"(error in=w282) -> (error out=w283:errorcluster, "TopLeft"=w284:T15)  [unwired: 1 in, 1 out]
        n123 = Select(t=w276, s=w275, f=0) -> (s? t:f=w277:i32)
        n124 = Bundle By Name(cluster=w284, "Row"=w277) -> (w285:T15)
        n125 = property on="多列列表框" class="MCListbox (严格)"(error in=w283, "TopLeft"=w285) -> ()  [unwired: 1 in, 2 out]
      }
    }
  }
  n126 = Build Path(base path=w7, name or relative path="data\\Set.ini" ("名称或相对路径")) -> (appended path=w5:path)
  n127 = timed-loop {
    timing: w17 -> [_]
    timing-out: [_] -> w16
    tunnel: w13 -> [w288]
    stop <- FALSE stop-if-true
    w289 = u16 3 items=["总磷"=1, "氨氮"=3] ("站号")
    # "定时更新"
    n128 = node-c288() -> ()  [unwired: 1 in, 1 out]
    n129 = call "总磷氨氮版本号读取.vi"() -> ("固件版本号"=→"固件版本号":string)  [unwired: 11 in]
    n130 = Bundle By Name(cluster=cluster{"命令":string, "data":variant} {"命令"="", "data"=variant} ("元素"), "命令"="读序列号", "data"=w289) -> (w287:cluster{"命令":string, "data":variant})
    n131 = Enqueue Element(queue=w288, element=w287) -> ()  [unwired: 2 in, 3 out]
    n132 = node-c288() -> ()  [unwired: 1 in, 1 out]
  }
  n133 = call <vilib>:"Open Config Data.vi"("configuration file path"=w5) -> ("error out"=w9:errorcluster, "refnum"=w11:T16)  [unwired: 8 in, 1 out]
  n134 = property class="VI"(reference=w43) -> ("Name"=w42:string)  [unwired: 1 in, 2 out]
  n135 = property class="VI"(reference=w35) -> ("Name"=w28:string)  [unwired: 1 in, 2 out]
  n136 = Open VI Reference(type specifier VI Refnum (for type only)=refnum<vi> refnum, vi path=w42, options=128 ("选项")) -> (vi reference=w40:refnum<vi>, error out=w38:errorcluster)  [unwired: 3 in]
  n137 = call-poly <vilib>:"Read Key.vi"("section"="总磷总氮", "error in (no error)"=w9, "key"="总氮稀释倍数" ("section"), "refnum"=w11) -> ("error out"=w8:errorcluster, "value"=→"总氮稀释倍数":dbl, "refnum out"=w10:T16)  [unwired: 4 in, 1 out]
  n138 = call-by-ref "?"(reference=w40, error in=w38) -> (reference out=w36:refnum<vi>, error out=w37:errorcluster)  [unwired: 12 in]
  n139 = Open VI Reference(type specifier VI Refnum (for type only)=refnum<vi> refnum, vi path=w28, options=128 ("选项")) -> (vi reference=w30:refnum<vi>, error out=w32:errorcluster)  [unwired: 3 in]
  n140 = call "时间延迟2"() -> ("error out"=w12:errorcluster)  [unwired: 11 in]
  n141 = call-by-ref "?"(reference=w30, error in=w32) -> (reference out=w34:refnum<vi>, error out=w33:errorcluster)  [unwired: 12 in]
  n142 = Close Reference(reference=w36, error in (no error)=w37) -> ()  [unwired: 1 out]
  n143 = Close Reference(reference=w34, error in (no error)=w33) -> ()  [unwired: 1 out]
  n144 = call "总磷氨氮MB_api.vi"("STEP"=enum16{"open", "read", "write", "close"}."open", "Error in"=w12) -> ("error out"=w19:errorcluster)  [unwired: 7 in, 2 out]
  n145 = call <vilib>:"Close Config Data.vi"("error in (no error)"=w8, "refnum"=w10) -> ("error out"=w3:errorcluster)  [unwired: 8 in, 1 out]
  n146 = control-ref of="测量模式下拉列表"() -> (w24:refnum<vi>)
  n147 = control-ref of="量程切换阈值"() -> (w22:refnum<vi>)
  n148 = control-ref of="参数下拉列表"() -> (w25:refnum<vi>)
  n149 = control-ref of="量程下拉列表"() -> (w26:refnum<vi>)
  n150 = node-c288(w16) -> ()  [unwired: 1 out]
  n151 = control-ref of="备用系数"() -> (w21:refnum<vi>)
  n152 = control-ref of="公式"() -> (w23:refnum<vi>)
  n153 = Obtain Queue(name (unnamed)="TP" ("名称（未命名）"), element data type=cluster{"命令":string, "data":variant} {"命令"="", "data"=variant}) -> (queue out=w46:refnum<queue>, error out=w47:errorcluster)  [unwired: 3 in, 1 out]
  n154 = while {
    tunnel: w46 -> [w298]
    shift-right: [w299] -> _
    shift-left: T4."待机" -> [w300]
    shift-right: [w296] -> _
    shift-left: u32 0 ("等待时间（毫秒）") -> [w297]
    stop <- FALSE stop-if-true
    n155 = Wait (ms)(milliseconds to wait=u32 1000 ("等待时间（毫秒）")) -> ()  [unwired: 1 out]
    n156 = local read "定时启动"() -> (w301:bool)
    n157 = case shown="真" w301 {
      tunnel: w300 -> [_ w310]
      tunnel: [T4."待机" w309] -> w299
      tunnel: w298 -> [_ w308]
      tunnel: w297 -> [_ w307]
      tunnel: [_ w306] -> w296
      tunnel: [_ w305] -> w295
      frame False {
      }
      frame True {
        n158 = case shown="\"总磷测量中\"" w310 {
          tunnel: [T4."启动氨氮" w317 w323 w337 w344 w363] -> w309
          tunnel: w308 -> [_ w322 _ w343 _ _]
          tunnel: w307 -> [_ _ _ _ _ w365]
          tunnel: [_ _ _ _ _ w357] -> w306
          tunnel: ["待机" ("字符串") "启动总氮" ("字符串") "总氮运行中" ("字符串") "启动总磷" ("字符串") "总磷运行中" ("字符串") w355] -> w305
          frame "待机", Default {
          }
          frame "启动氨氮" {
            n159 = call "总磷氨氮启动命令.vi"("参数"=T17 {"站号"=2, "量程切换"=enum."AUTO", "控制命令"=enum."启动测量", "模式设置"=enum."待机", "测量间隔"=0}) -> ("启动命令"=w315:cluster{"命令":string, "data":variant})  [unwired: 10 in]
            n160 = Enqueue Element(queue=w322, element=w315) -> ()  [unwired: 2 in, 3 out]
            n161 = global read "VAR总磷氨氮全局变量.vi" "状态告警区"() -> (w321:T3)
            n162 = Unbundle By Name(w321) -> ("工作状态"=w320:T7)
            n163 = Not Equal To 0?(x=w320) -> (x != 0?=w319:bool)
            n164 = Select(t=T4."氨氮测量中", s=w319, f=T4."启动氨氮") -> (s? t:f=w317:T4)
          }
          frame "氨氮测量中" {
            n165 = global read "VAR总磷氨氮全局变量.vi" "状态告警区"() -> (w326:T3)
            n166 = Unbundle By Name(w326) -> ("工作状态"=w324:T7, "id"=w325:u16)
            n167 = case shown="默认" w324 {
              tunnel: w325 -> [_ w331]
              tunnel: [T4."启动总磷" w330] -> w323
              frame "空闲" {
                n168 = Wait (ms)(milliseconds to wait=u32 8000 ("等待时间（毫秒）")) -> ()  [unwired: 1 out]
              }
              frame Default {
                n169 = case shown="76, 默认" w331 {
                  tunnel: [T4."氨氮测量中" T4."总磷测量中"] -> w330
                  frame 76, Default {
                  }
                  frame 131 {
                  }
                }
              }
            }
          }
          frame "启动总磷" {
            n170 = call "总磷氨氮启动命令.vi"("参数"=T17 {"站号"=1, "量程切换"=enum."AUTO", "控制命令"=enum."启动测量", "模式设置"=enum."待机", "测量间隔"=0}) -> ("启动命令"=w336:cluster{"命令":string, "data":variant})  [unwired: 10 in]
            n171 = Enqueue Element(queue=w343, element=w336) -> ()  [unwired: 2 in, 3 out]
            n172 = global read "VAR总磷氨氮全局变量.vi" "状态告警区"() -> (w338:T3)
            n173 = Unbundle By Name(w338) -> ("工作状态"=w339:T7)
            n174 = Not Equal To 0?(x=w339) -> (x != 0?=w340:bool)
            n175 = Select(t=T4."总磷测量中", s=w340, f=T4."启动总磷") -> (s? t:f=w337:T4)
          }
          frame "总磷测量中" {
            n176 = global read "VAR总磷氨氮全局变量.vi" "状态告警区"() -> (w347:T3)
            n177 = Unbundle By Name(w347) -> ("工作状态"=w345:T7, "id"=w346:u16)
            n178 = case shown="默认" w345 {
              tunnel: w346 -> [_ w352]
              tunnel: [T4."延时" w351] -> w344
              frame "空闲" {
                n179 = Wait (ms)(milliseconds to wait=u32 8000 ("等待时间（毫秒）")) -> ()  [unwired: 1 out]
              }
              frame Default {
                n180 = case shown="76, 默认" w352 {
                  tunnel: [T4."氨氮测量中" T4."总磷测量中"] -> w351
                  frame 76, Default {
                  }
                  frame 131 {
                  }
                }
              }
            }
          }
          frame "延时" {
            n181 = local read "设置值"() -> (w360:dbl)
            n182 = Increment(x=w365) -> (x+1=w357:u32)
            n183 = Add(x=w360, y=10.0) -> (x+y=w358:dbl)
            n184 = Greater Or Equal?(x=w357, y=w358) -> (x >= y?=w364:bool)
            n185 = Select(t=T4."待机", s=w364, f=T4."延时") -> (s? t:f=w363:T4)
            n186 = Format Into String(format string="延时计时中%d秒" ("格式字符串"), w357) -> (resulting string=w355:string)  [unwired: 2 in, 1 out]
          }
        }
      }
    }
    "字符串" <- w295
  }
  n187 = while {
    tunnel: w46 -> [w373]
    tunnel: w26 -> [w372]
    tunnel: w25 -> [w371]
    tunnel: w24 -> [w370]
    tunnel: w23 -> [w369]
    tunnel: w22 -> [w368]
    tunnel: w21 -> [w367]
    tunnel: w19 -> [_]
    tunnel: w3 -> [w366]
    stop <- FALSE stop-if-true
    n188 = event shown="[15] \"总氮稀释倍数\": 值改变" {
      selector: _ -> [_ _ _ _ _ _ _ _ _ _ _ _ _ _ _ _]
      dyn-events: _ -> [_ _ _ _ _ _ _ _ _ _ _ _ _ _ _ _]
      timeout: _ -> [_ _ _ _ _ _ _ _ _ _ _ _ _ _ _ _]
      tunnel: w373 -> [_ w377 _ w388 w390 _ _ _ _ _ _ _ _ _ _ _]
      tunnel: w372 -> [_ _ _ _ _ _ _ _ _ w443 _ w463 w472 _ _ _]
      tunnel: w371 -> [_ _ _ _ _ _ _ _ _ w441 _ w461 w474 w482 w489 _]
      tunnel: w370 -> [_ _ _ _ _ _ _ _ _ w442 _ w462 w473 _ _ _]
      tunnel: w369 -> [_ _ _ _ _ _ _ _ _ w437 _ _ _ _ _ _]
      tunnel: w368 -> [_ _ _ _ _ _ _ _ _ _ _ w457 _ _ _ _]
      tunnel: w367 -> [_ _ _ _ _ _ _ _ _ _ _ _ _ w480 _ _]
      tunnel: w366 -> [_ _ _ _ _ _ _ _ _ _ _ _ _ _ _ _]
      event Timeout {
        n189 = event-data() -> ()  [unwired: 1 in, 3 out]
      }
      event "手动启动": Value Change {
        n190 = event-data() -> ()  [unwired: 1 in, 6 out]
        n191 = call "总磷氨氮启动参数对话框.vi"() -> ("确认"=w375:bool, "元素"=w376:cluster{"命令":string, "data":variant})  [unwired: 10 in]
        n192 = case shown="真" w375 {
          tunnel: w377 -> [_ w379]
          tunnel: w376 -> [_ w378]
          frame False {
          }
          frame True {
            n193 = Enqueue Element(queue=w379, element=w378) -> ()  [unwired: 2 in, 3 out]
          }
        }
      }
      event "定时启动": Mouse Down {
        n194 = event-data() -> ()  [unwired: 1 in, 6 out]
        n195 = call "定时启动对话框.vi"() -> ("设置值"=→"设置值":dbl, "确定输出"=→"定时启动":bool)  [unwired: 10 in]
      }
      event "单步测试": Value Change {
        w383 = u16 1 items=["总磷"=1, "氨氮"=3] ("站号")
        n196 = event-data() -> ()  [unwired: 1 in, 6 out]
        n197 = Bundle("站号"=w383, "总磷氨氮调试"="总磷氨氮调试") -> (w382:cluster{"站号":u16, "总磷氨氮调试":u16[]})  [unwired: 1 in]
        n198 = Bundle By Name(cluster=cluster{"命令":string, "data":variant} {"命令"="", "data"=variant} ("元素"), "命令"="debug", "data"=w382) -> (w385:cluster{"命令":string, "data":variant})
        n199 = Enqueue Element(queue=w388, element=w385) -> ()  [unwired: 2 in, 3 out]
      }
      event "停止": Value Change {
        n200 = event-data() -> ()  [unwired: 1 in, 6 out]
        n201 = Enqueue Element(queue=w390, element=cluster{"命令":string, "data":variant} {"命令"="启动", "data"=variant(cluster{"站号":u16, "控制命令输出":u16[]} {"站号"=1, "控制命令输出"=[2816]})} ("元素")) -> ()  [unwired: 2 in, 3 out]
      }
      event "设置": Value Change {
        n202 = event-data() -> ()  [unwired: 1 in, 6 out]
        n203 = property on="窗格" class="Pane"("Origin"=T5 {"Horizontal"=0, "Vertical"=628} ("原点")) -> ()  [unwired: 2 in, 2 out]
      }
      event "返回": Value Change {
        n204 = event-data() -> ()  [unwired: 1 in, 6 out]
        n205 = property on="窗格" class="Pane"("Origin"=T5 {"Horizontal"=0, "Vertical"=0} ("原点")) -> ()  [unwired: 2 in, 2 out]
      }
      event "标液浓度1", "测量吸光度1", "测量吸光度2", "标液浓度2", "测量吸光度3", "标液浓度3", "测量吸光度4", "标液浓度4", "测量吸光度5", "标液浓度5", "样品1启用", "样品3启用", "样品4启用", "样品5启用", "样品2启用", "模型", "method", "样品1 F0", "样品1 F1", "样品2 F1", "样品2 F0", "样品3 F1", "样品4 F0", "样品4 F1", "样品5 F1", "样品5 F0", "精度": Value Change {
        n206 = event-data() -> ()  [unwired: 1 in, 6 out]
        n207 = formula code="E=log(F0/F1);"("F0"="样品1 F0", "F1"="样品1 F1") -> ("E"=w414:dbl)
        "测量吸光度1" <- w414
        n208 = formula code="E=log(F0/F1);"("F0"="样品2 F0", "F1"="样品2 F1") -> ("E"=w411:dbl)
        "测量吸光度2" <- w411
        n209 = formula code="E=log(F0/F1);"("F0"="样品3 F0", "F1"="样品3 F1") -> ("E"=w408:dbl)
        "测量吸光度3" <- w408
        n210 = formula code="E=log(F0/F1);"("F0"="样品4 F0", "F1"="样品4 F1") -> ("E"=w405:dbl)
        "测量吸光度4" <- w405
        n211 = formula code="E=log(F0/F1);"("F0"="样品5 F0", "F1"="样品5 F1") -> ("E"=w402:dbl)
        "测量吸光度5" <- w402
        n212 = Replace Array Subset(array=dbl[] [0.0, 0.0, 0.0, 0.0, 0.0] ("数组"), new element #1="标液浓度1", new element #2="标液浓度2", new element #3="标液浓度3", new element #4="标液浓度4", new element #5="标液浓度5") -> (w399:dbl[])  [unwired: 5 in]
        n213 = Replace Array Subset(array=dbl[] [0.0, 0.0, 0.0, 0.0, 0.0] ("数组"), new element #1=w414, new element #2=w411, new element #3=w408, new element #4=w405, new element #5=w402) -> (w398:dbl[])  [unwired: 5 in]
        n214 = Replace Array Subset(array=bool[] [FALSE, FALSE, FALSE, FALSE, FALSE] ("数组"), new element #1="样品1启用", new element #2="样品2启用", new element #3="样品3启用", new element #4="样品4启用", new element #5="样品5启用") -> (w397:bool[])  [unwired: 5 in]
        n215 = call "线性公式.vi"("精度"="精度", "模型"="模型", "method"="method", "启用"=w397, "监测浓度"=w398, "标液浓度"=w399) -> ("XY图"=→"XY图":cluster{"X Values":dbl[], "Y Values":dbl[]}[], "r^2"=→"r^2":dbl, "拟合方程"=→"拟合公式":string)  [unwired: 3 in]
      }
      event "标液浓度1", "标液浓度2", "标液浓度3", "标液浓度4", "标液浓度5", "样品1 F0", "样品1 F1", "样品2 F1", "样品2 F0", "样品3 F1", "样品3 F0", "样品4 F0", "样品4 F1", "样品5 F0", "样品5 F1", "精度", "公式.X^2", "公式.X", "公式.b", "量程切换阈值.阈值", "量程切换阈值.标液浓度", "备用系数.量程上限", "备用系数.量程下限", "备用系数.检出限", "备用系数.精度", "总氮稀释倍数": Mouse Down {
        n216 = event-data() -> ("CtlRef"=w433:refnum<vi>)  [unwired: 1 in, 5 out]
        n217 = property class="DigNum (严格)"(reference=w433) -> (reference out=w431:refnum<vi>, "Value"=w432:dbl)  [unwired: 1 in, 1 out]
        n218 = call "数字键盘.vi"("OldNumber"=w432) -> ("NewNumber"=w430:sgl)
        n219 = property class="DigNum (严格)"(reference=w431, "Val(Sgnl)"=w430) -> ()  [unwired: 1 in, 2 out]
      }
      event "读公式": Value Change {
        n220 = event-data() -> ()  [unwired: 1 in, 6 out]
        n221 = property class="Enum (严格)"(reference=w441) -> ("Value"=w440:enum16{"总磷", "总氮"})  [unwired: 1 in, 2 out]
        n222 = property class="Enum (严格)"(reference=w442) -> ("Value"=w439:enum16{"水样测量", "空白核查", "跨度核查", "标样核查", "加标回收"})  [unwired: 1 in, 2 out]
        n223 = property class="Enum (严格)"(reference=w443) -> ("Value"=w438:enum16{"低量程", "高量程"})  [unwired: 1 in, 2 out]
        n224 = call "总磷氨氮公式读取.vi"("量程"=w438, "测量模式"=w439, "测量参数"=w440) -> ("error out"=w435:errorcluster, "公式"=w436:cluster{"X^2":dbl, "X":dbl, "b":dbl})  [unwired: 7 in]
        n225 = property class="Clust (严格)"(reference=w437, "Value"=w436) -> ()  [unwired: 1 in, 2 out]
        n226 = case shown="错误" w435 {
          tunnel: ["读取成功" ("消息") "读取失败" ("消息")] -> w434
          frame No Error {
          }
          frame Error {
          }
        }
        n227 = One Button Dialog(message=w434) -> ()  [unwired: 1 in, 1 out]
      }
      event "写公式": Value Change {
        n228 = event-data() -> ()  [unwired: 1 in, 6 out]
        n229 = call "总磷氨氮公式写入.vi"("公式"="公式", "量程"="量程下拉列表", "测量模式"="测量模式下拉列表", "测量参数"="参数下拉列表") -> ("error out"=w448:errorcluster)  [unwired: 7 in]
        n230 = case shown="无错误" w448 {
          tunnel: ["写入成功" ("消息") "写入失败" ("消息")] -> w449
          frame No Error {
          }
          frame Error {
          }
        }
        n231 = One Button Dialog(message=w449) -> ()  [unwired: 1 in, 1 out]
      }
      event "量程切换阈值读取": Value Change {
        n232 = event-data() -> ()  [unwired: 1 in, 6 out]
        n233 = property class="Enum (严格)"(reference=w461) -> ("Value"=w460:enum16{"总磷", "总氮"})  [unwired: 1 in, 2 out]
        n234 = property class="Enum (严格)"(reference=w462) -> ("Value"=w459:enum16{"水样测量", "空白核查", "跨度核查", "标样核查", "加标回收"})  [unwired: 1 in, 2 out]
        n235 = property class="Enum (严格)"(reference=w463) -> ("Value"=w458:enum16{"低量程", "高量程"})  [unwired: 1 in, 2 out]
        n236 = call "总磷氨氮量程读取.vi"("量程"=w458, "测量模式"=w459, "测量参数"=w460) -> ("error out"=w454:errorcluster, "量程切换阈值"=w456:cluster{"阈值":dbl, "标液浓度":dbl})  [unwired: 7 in]
        n237 = property class="Clust (严格)"(reference=w457, "Value"=w456) -> ()  [unwired: 1 in, 2 out]
        n238 = case shown="错误" w454 {
          tunnel: ["读取成功" ("消息") "读取失败" ("消息")] -> w455
          frame No Error {
          }
          frame Error {
          }
        }
        n239 = One Button Dialog(message=w455) -> ()  [unwired: 1 in, 1 out]
      }
      event "量程切换阈值写入": Value Change {
        n240 = event-data() -> ()  [unwired: 1 in, 6 out]
        n241 = property class="Enum (严格)"(reference=w474) -> ("Value"=w471:enum16{"总磷", "总氮"})  [unwired: 1 in, 2 out]
        n242 = property class="Enum (严格)"(reference=w473) -> ("Value"=w470:enum16{"水样测量", "空白核查", "跨度核查", "标样核查", "加标回收"})  [unwired: 1 in, 2 out]
        n243 = property class="Enum (严格)"(reference=w472) -> ("Value"=w469:enum16{"低量程", "高量程"})  [unwired: 1 in, 2 out]
        n244 = call "总磷氨氮量程写入.vi"("量程切换阈值"="量程切换阈值", "量程"=w469, "测量模式"=w470, "测量参数"=w471) -> ("error out"=w466:errorcluster)  [unwired: 7 in]
        n245 = case shown="无错误" w466 {
          tunnel: ["写入成功" ("消息") "写入失败" ("消息")] -> w467
          frame No Error {
          }
          frame Error {
          }
        }
        n246 = One Button Dialog(message=w467) -> ()  [unwired: 1 in, 1 out]
      }
      event "备用系数读取": Value Change {
        n247 = event-data() -> ()  [unwired: 1 in, 6 out]
        n248 = property class="Enum (严格)"(reference=w482) -> ("Value"=w481:enum16{"总磷", "总氮"})  [unwired: 1 in, 2 out]
        n249 = call "总磷氨氮备用系数读取.vi"("测量参数"=w481) -> ("error out"=w477:errorcluster, "备用系数"=w479:T1)  [unwired: 9 in]
        n250 = property class="Clust (严格)"(reference=w480, "Value"=w479) -> ()  [unwired: 1 in, 2 out]
        n251 = case shown="错误" w477 {
          tunnel: ["读取成功" ("消息") "读取失败" ("消息")] -> w478
          frame No Error {
          }
          frame Error {
          }
        }
        n252 = One Button Dialog(message=w478) -> ()  [unwired: 1 in, 1 out]
      }
      event "备用系数写入": Value Change {
        n253 = event-data() -> ()  [unwired: 1 in, 6 out]
        n254 = property class="Enum (严格)"(reference=w489) -> ("Value"=w488:enum16{"总磷", "总氮"})  [unwired: 1 in, 2 out]
        n255 = call "总磷氨氮备用系数写入.vi"("备用系数"="备用系数", "测量参数"=w488) -> ("error out"=w485:errorcluster)  [unwired: 9 in]
        n256 = case shown="无错误" w485 {
          tunnel: ["写入成功" ("消息") "写入失败" ("消息")] -> w486
          frame No Error {
          }
          frame Error {
          }
        }
        n257 = One Button Dialog(message=w486) -> ()  [unwired: 1 in, 1 out]
      }
      event "总氮稀释倍数": Value Change {
        n258 = event-data() -> ()  [unwired: 1 in, 6 out]
        n259 = call <vilib>:"Application Directory.vi"() -> ("Application Directory"=w499:path)
        n260 = Build Path(base path=w499, name or relative path="data\\Set.ini" ("名称或相对路径")) -> (appended path=w501:path)
        n261 = local read "总氮稀释倍数"() -> (w494:dbl)
        n262 = call <vilib>:"Open Config Data.vi"("configuration file path"=w501) -> ("error out"=w496:errorcluster, "refnum"=w498:T16)  [unwired: 8 in, 1 out]
        n263 = global write "VAR总磷氨氮全局变量.vi" "总氮稀释倍数"(w494) -> ()
        n264 = call-poly <vilib>:"Write Key.vi"("section"="总磷总氮", "error in (no error)"=w496, "value"=w494, "key"="总氮稀释倍数" ("section"), "refnum"=w498) -> ("error out"=w495:errorcluster, "refnum out"=w497:T16)  [unwired: 4 in, 1 out]
        n265 = call <vilib>:"Close Config Data.vi"("error in (no error)"=w495, "refnum"=w497) -> ()  [unwired: 8 in, 2 out]
      }
    }
  }
  n266 = while {
    tunnel: w46 -> [w518]
    tunnel: w47 -> [_]
    shift-right: [w510] -> _
    shift-left: enum16{"总磷", "总氮"}."总磷" ("枚举") -> [w512]
    stop <- FALSE stop-if-true
    # "试剂填充 172 \n管路清洗108\n氨氮92\n总磷131\n总磷海水147\n总氮76\n总氮海水92"
    n267 = case shown="\"总氮\", 默认" w512 {
      selector: w512 -> [w527 w529]
      tunnel: [w528 w530] -> w513
      tunnel: [w527 w529] -> w511
      frame "总氮", Default {
        w528 = u16 2 items=["总磷"=1, "总氮"=2] ("站号")
      }
      frame "总磷" {
        w530 = u16 1 items=["总磷"=1, "氨氮"=3] ("站号")
      }
    }
    n268 = Wait (ms)(milliseconds to wait=u32 1000 ("等待时间（毫秒）")) -> ()  [unwired: 1 out]
    n269 = Bundle By Name(cluster=cluster{"命令":string, "data":variant} {"命令"="", "data"=variant} ("元素"), "命令"="读状态告警区", "data"=w513) -> (w520:cluster{"命令":string, "data":variant})
    n270 = global read "VAR总磷氨氮全局变量.vi" "状态告警区"() -> (w502:T3)
    n271 = Unbundle By Name(w502) -> ("系统时间"=w509:timestamp)
    n272 = Enqueue Element(queue=w518, element=w520) -> (queue out=w514:refnum<queue>)  [unwired: 2 in, 2 out]
    n273 = Get Date/Time In Seconds() -> (seconds since 1Jan1904=w508:timestamp)
    n274 = Subtract(x=w508, y=w509) -> (x-y=w507:dbl)
    n275 = Bundle By Name(cluster=cluster{"命令":string, "data":variant} {"命令"="", "data"=variant} ("元素"), "命令"="读测量数据区", "data"=w513) -> (w516:cluster{"命令":string, "data":variant})
    n276 = Absolute Value(x=w507) -> (abs(x)=w506:dbl)
    n277 = Enqueue Element(queue=w514, element=w516) -> (queue out=w503:refnum<queue>)  [unwired: 2 in, 2 out]
    n278 = Greater Or Equal?(x=w506, y=120.0) -> (x >= y?=w504:bool)
    n279 = case shown="真" w504 {
      tunnel: w503 -> [_ w525]
      frame False {
      }
      frame True {
        n280 = call "总磷氨氮启动命令.vi"("参数"=T18 {"站号"=3, "量程切换"=enum."AUTO", "控制命令"=enum."校时", "模式设置"=enum."待机", "测量间隔"=0}) -> ("启动命令"=w524:cluster{"命令":string, "data":variant})  [unwired: 10 in]
        n281 = Enqueue Element(queue=w525, element=w524) -> ()  [unwired: 2 in, 3 out]
      }
    }
    n282 = Increment(x=w511) -> (x+1=w510:enum16{"总磷", "总氮"})
  }
